vi "Update VS channels - outgoing (interaction info).vi"(8 "interaction info":T5, 9 "interaction handle":u64, 10 "out_interactionMap in":T6, 11 "values in":dbl[](array[numeric])) -> (2 "out_interactionMap out":T6, 3 "values out":dbl[](array[numeric]))   [LabVIEW 2019, in "HLA Custom Device Engine.lvlib"]
uses:
  HLA Custom Device Engine.lvlib
  _typedefs/map_in_interaction.ctl
  _typedefs/map_interaction_value.ctl
  _typedefs/map_attr_param_data.ctl
  _typedefs/interaction_info_outgoing_type.ctl
  _typedefs/map_object.ctl
  _typedefs/map_object_key.ctl
  _typedefs/map_object_value.ctl
panel:
  in  "runtime data.hlaMap.out_objectMap":T1
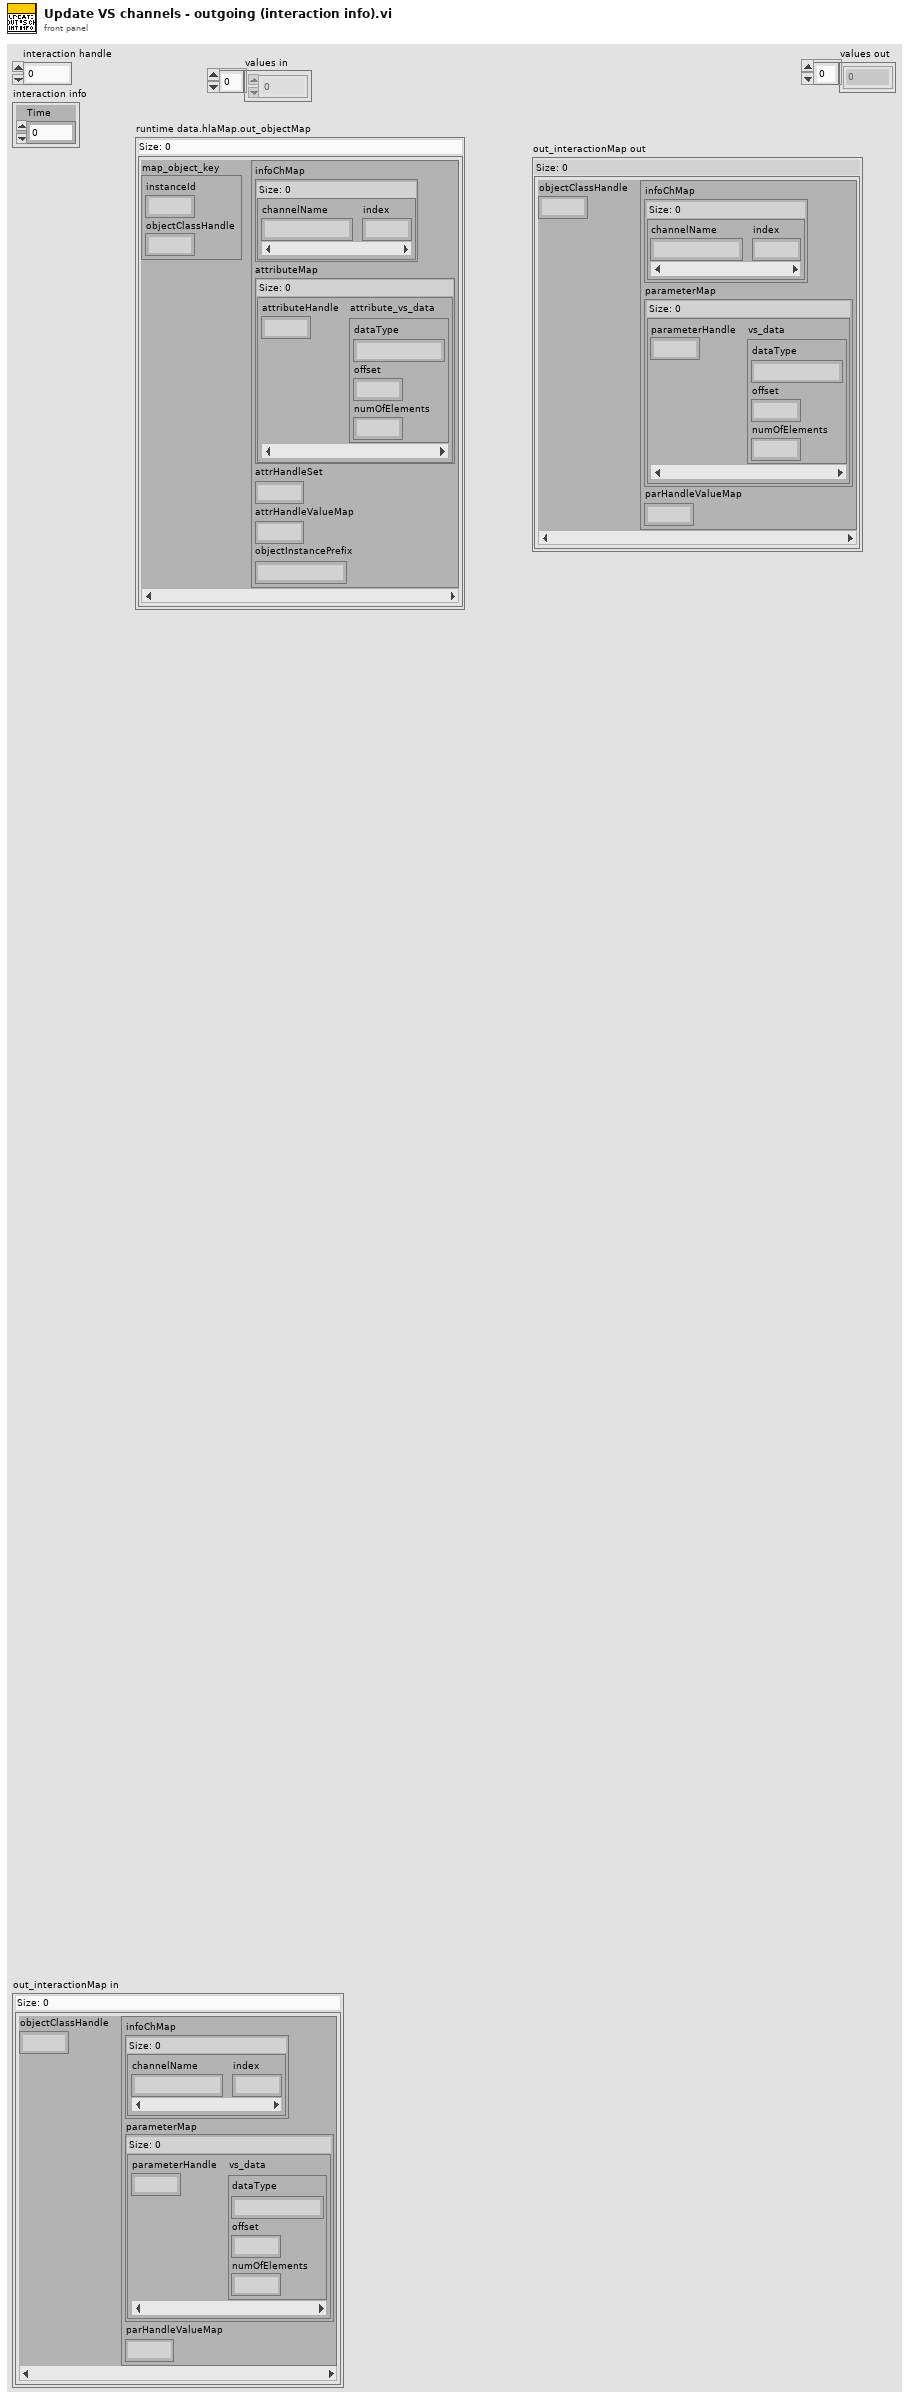
[diagram p1: front panel]
types:
  T1 = typedef "HLA Custom Device Engine.lvlib/map_object.ctl" = map{T2, T3}
  T2 = typedef "HLA Custom Device Engine.lvlib/map_object_key.ctl" = cluster{"instanceId":i32, "objectClassHandle":u64}
  T3 = typedef "HLA Custom Device Engine.lvlib/map_object_value.ctl" = cluster{"infoChMap":map{string, i32}, "attributeMap":map{u64, T4}, "attrHandleSet":u64, "attrHandleValueMap":u64, "objectInstancePrefix":string}
  T4 = typedef "HLA Custom Device Engine.lvlib/map_attr_param_data.ctl" = cluster{"dataType":string, "offset":i32, "numOfElements":i32}
  T5 = typedef "HLA Custom Device Engine.lvlib/interaction_info_outgoing_type.ctl" = cluster{"Time":dbl}
  T6 = typedef "HLA Custom Device Engine.lvlib/map_in_interaction.ctl" = map{u64, T7}
  T7 = typedef "HLA Custom Device Engine.lvlib/map_interaction_value.ctl" = cluster{"infoChMap":map{string, i32}, "parameterMap":map{u64, T4}, "parHandleValueMap":u64}
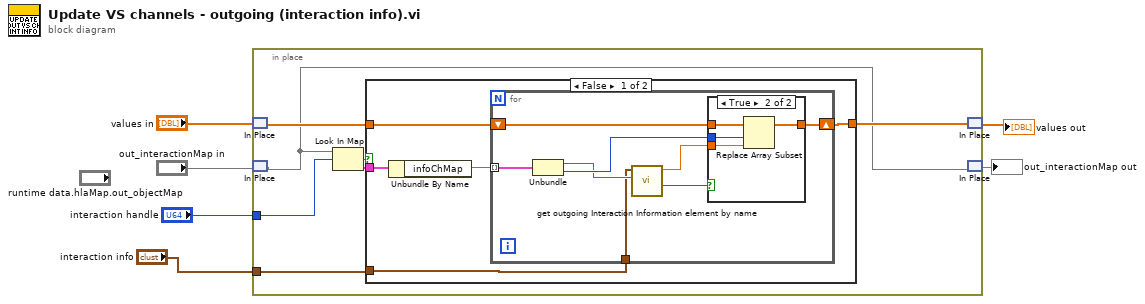
[diagram p0: block diagram]
diagram:
  n1 = in-place {
    in-place-border: "interaction handle" -> [w8]
    in-place-border: "interaction info" -> [w7]
    n2 = in-place-match #1("values in") -> (w11:dbl[])
    n3 = in-place-match #2("out_interactionMap in") -> (w9:T6)
    n4 = Look In Map(map=w9, key=w8) -> (key not found?=w13:bool, value=w12:T7)  [unwired: 1 in]
    n5 = case shown="False" w13 {
      tunnel: [w17 w32] -> w10
      tunnel: w12 -> [w15 _]
      tunnel: w11 -> [w16 w32]
      tunnel: w7 -> [w14 _]
      frame False {
        n6 = Unbundle By Name(w15) -> ("infoChMap"=w18:map{string, i32})
        n7 = for {
          tunnel: w18 -> [w23] mode=indexing
          shift-right: [w25] -> w17
          shift-left: w16 -> [w26]
          tunnel: w14 -> [w19]
          n8 = Unbundle(w23) -> ("channelName"=w22:string, "index"=w24:i32)
          n9 = call "get outgoing Interaction Information element by name.vi"("name"=w22, "interaction_attribute_type"=w19) -> ("found"=w20:bool, "element out"=w21:dbl)  [unwired: 8 in]
          n10 = case shown="True" w20 {
            tunnel: w26 -> [w27 w31]
            tunnel: [w27 w30] -> w25
            tunnel: w21 -> [_ w29]
            tunnel: w24 -> [_ w28]
            frame False {
            }
            frame True {
              n11 = Replace Array Subset(array=w31, new element=w29, index=w28) -> (w30:dbl[])
            }
          }
        }
      }
      frame True {
      }
    }
    n12 = in-place-match #1(w10) -> (→"values out":dbl[])
    n13 = in-place-match #2(w9) -> (→"out_interactionMap out":T6)
  }
